vi "ArrangeFrontPanel.vi"(8 "error in (no error)":errorcluster, 10 "This VI":refnum<vi>, 11 "MAUI in":refnum<class "MAUI.lvclass">) -> (0 "error out":errorcluster, 3 "MAUI out":refnum<class "MAUI.lvclass">)   [LabVIEW 2019, in "MAUI.lvclass"]
doc: "This VI is mainly used for the MAUI Template. It will be removed from the library soon."
uses:
  MAUI.lvclass
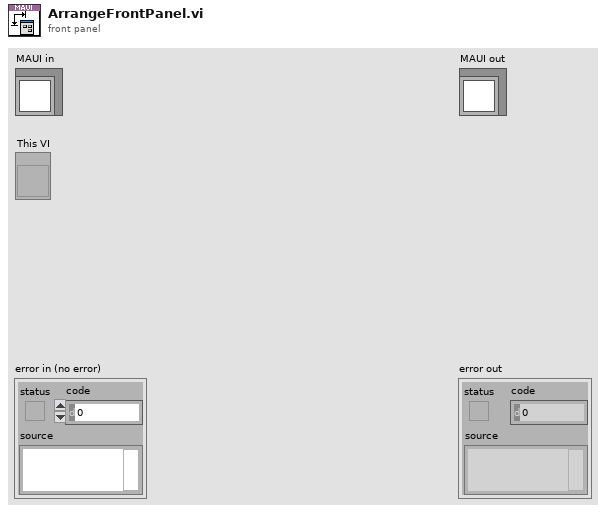
[diagram p1: front panel]
types:
  T1 = typedef "LVRectTypeDef.ctl" = cluster{"Left":i16, "Top":i16, "Right":i16, "Bottom":i16}
  T2 = typedef "LVBoundsTypeDef.ctl" = cluster{"Width":u32, "Height":u32}
  T3 = enum16{"Always On", "Always Off", "Off While Running"}
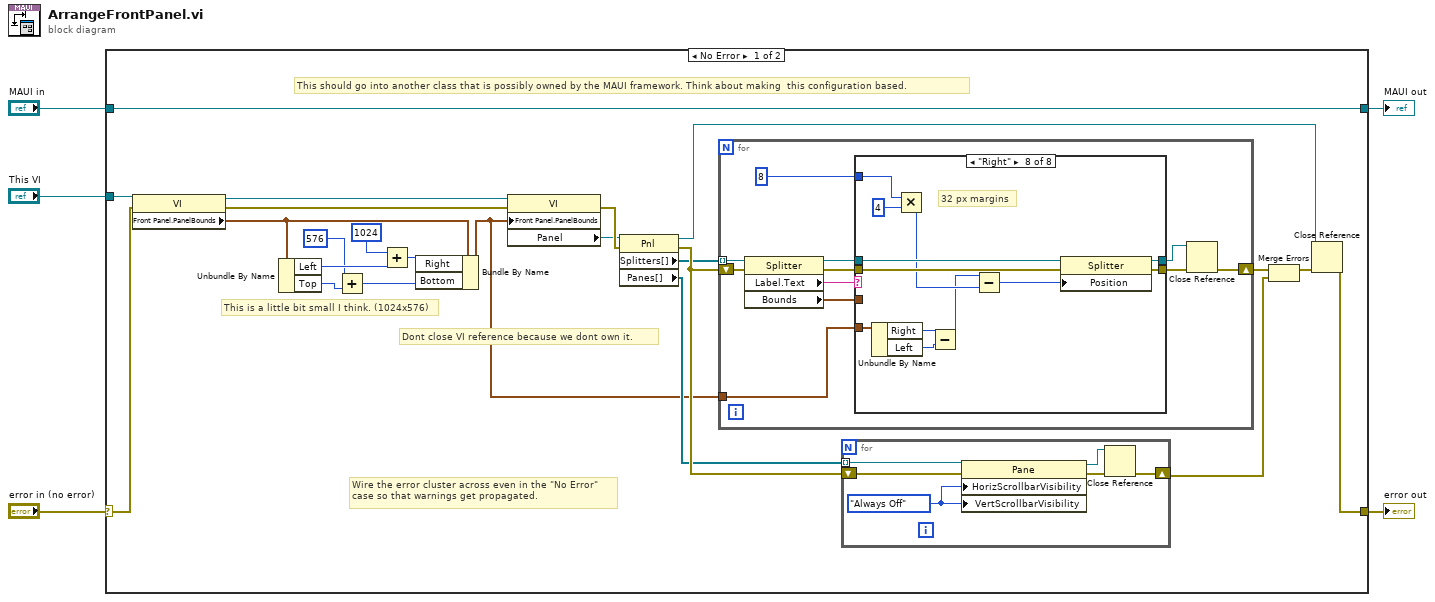
[diagram p0: block diagram]
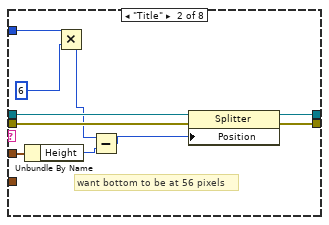
[diagram p3: hidden frame]
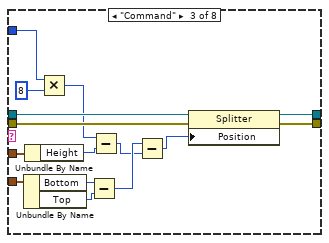
[diagram p4: hidden frame]
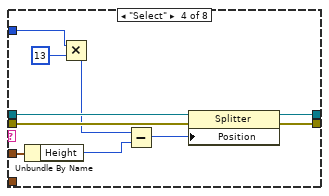
[diagram p5: hidden frame]
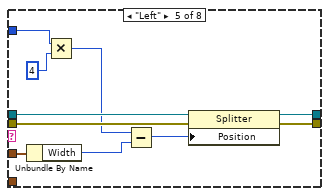
[diagram p6: hidden frame]
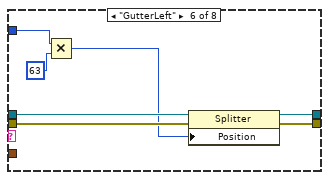
[diagram p7: hidden frame]
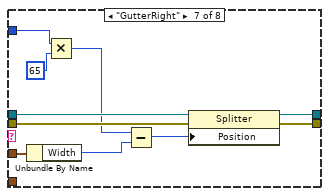
[diagram p8: hidden frame]
diagram:
  n1 = case shown="No Error" "error in (no error)" {
    selector: "error in (no error)" -> [w26 w123]
    tunnel: [w25 w123] -> w4
    tunnel: [w20 w122] -> w2
    tunnel: "MAUI in" -> [w20 w122]
    tunnel: "This VI" -> [w19 _]
    frame No Error {
      # "This should go into another class that is possibly owned by the MAUI framework. Think about making  this configuration based."
      # "This is a little bit small I think. (1024x576)"
      # "Dont close VI reference because we dont own it."
      # "Wire the error cluster across even in the \"No Error\"\ncase so that warnings get propagated."
      n2 = property on="Property Node" class="VI"(reference=w19, error in=w26) -> (reference out=w14:refnum<vi>, error out=w28:errorcluster, "Front Panel.PanelBounds"=w18:T1)
      n3 = Unbundle By Name(w18) -> ("Left"=w16:i16, "Top"=w7:i16)
      n4 = Add(x=i16 576, y=w7) -> (x+y=w17:i16)
      n5 = Add(x=i16 1024, y=w16) -> (x+y=w15:i16)
      n6 = Bundle By Name(cluster=w18, "Right"=w15, "Bottom"=w17) -> (w8:T1)
      n7 = property on="Property Node" class="VI"(reference=w14, error in=w28, "Front Panel.PanelBounds"=w8) -> (error out=w27:errorcluster, "Panel"=w13:refnum<vi>)  [unwired: 1 out]
      n8 = property on="Property Node" class="Pnl"(reference=w13, error in=w27) -> (reference out=w11:refnum<vi>, error out=w24:errorcluster, "Splitters[]"=w12:refnum<vi>[], "Panes[]"=w10:refnum<vi>[])
      n9 = for {
        tunnel: w12 -> [w41] mode=indexing
        shift-right: [w43] -> w23
        shift-left: w24 -> [w45]
        tunnel: w8 -> [w35]
        n10 = property on="Property Node" class="Splitter"(reference=w41, error in=w45) -> (reference out=w38:refnum<vi>, error out=w44:errorcluster, "Label.Text"=w40:string, "Bounds"=w39:T2)
        n11 = case shown="\"Right\"" w40 {
          tunnel: w44 -> [w47 w57 w72 w82 w92 w99 w109 w120]
          tunnel: w39 -> [_ w54 w69 w79 w89 _ w106 _]
          tunnel: [w47 w56 w71 w81 w91 w98 w108 w121] -> w42
          tunnel: w38 -> [w46 w55 w70 w80 w90 w97 w107 w118]
          tunnel: [w46 w51 w66 w77 w87 w96 w104 w119] -> w37
          tunnel: 8 -> [_ w50 w65 w75 w85 w95 w102 w117]
          tunnel: w35 -> [_ _ w63 _ _ _ _ w115]
          frame Default {
          }
          frame "Title" {
            # "want bottom to be at 56 pixels"
            n12 = Unbundle By Name(w54) -> ("Height"=w53:u32)
            n13 = Multiply(x=w50, y=6) -> (x*y=w48:i32)
            n14 = Subtract(x=w48, y=w53) -> (x-y=w52:u32)
            n15 = property on="Property Node" class="Splitter"(reference=w55, error in=w57, "Position"=w52) -> (reference out=w51:refnum<vi>, error out=w56:errorcluster)
          }
          frame "Command" {
            n16 = Unbundle By Name(w63) -> ("Bottom"=w62:i16, "Top"=w61:i16)
            n17 = Unbundle By Name(w69) -> ("Height"=w68:u32)
            n18 = Multiply(x=w65, y=8) -> (x*y=w67:i32)
            n19 = Subtract(x=w62, y=w61) -> (x-y=w59:i16)
            n20 = Subtract(x=w67, y=w68) -> (x-y=w58:u32)
            n21 = Subtract(x=w59, y=w58) -> (x-y=w60:u32)
            n22 = property on="Property Node" class="Splitter"(reference=w70, error in=w72, "Position"=w60) -> (reference out=w66:refnum<vi>, error out=w71:errorcluster)
          }
          frame "Select" {
            n23 = Unbundle By Name(w79) -> ("Height"=w76:u32)
            n24 = Multiply(x=w75, y=13) -> (x*y=w73:i32)
            n25 = Subtract(x=w73, y=w76) -> (x-y=w78:u32)
            n26 = property on="Property Node" class="Splitter"(reference=w80, error in=w82, "Position"=w78) -> (reference out=w77:refnum<vi>, error out=w81:errorcluster)
          }
          frame "Left" {
            n27 = Unbundle By Name(w89) -> ("Width"=w86:u32)
            n28 = Multiply(x=w85, y=4) -> (x*y=w83:i32)
            n29 = Subtract(x=w83, y=w86) -> (x-y=w88:u32)
            n30 = property on="Property Node" class="Splitter"(reference=w90, error in=w92, "Position"=w88) -> (reference out=w87:refnum<vi>, error out=w91:errorcluster)
          }
          frame "GutterLeft" {
            n31 = Multiply(x=w95, y=63) -> (x*y=w93:i32)
            n32 = property on="Property Node" class="Splitter"(reference=w97, error in=w99, "Position"=w93) -> (reference out=w96:refnum<vi>, error out=w98:errorcluster)
          }
          frame "GutterRight" {
            n33 = Unbundle By Name(w106) -> ("Width"=w103:u32)
            n34 = Multiply(x=w102, y=65) -> (x*y=w100:i32)
            n35 = Subtract(x=w100, y=w103) -> (x-y=w105:u32)
            n36 = property on="Property Node" class="Splitter"(reference=w107, error in=w109, "Position"=w105) -> (reference out=w104:refnum<vi>, error out=w108:errorcluster)
          }
          frame "Right" {
            # "32 px margins"
            n37 = Unbundle By Name(w115) -> ("Right"=w114:i16, "Left"=w113:i16)
            n38 = Multiply(x=w117, y=4) -> (x*y=w112:i32)
            n39 = Subtract(x=w114, y=w113) -> (x-y=w111:i16)
            n40 = Subtract(x=w111, y=w112) -> (x-y=w110:i32)
            n41 = property on="Property Node" class="Splitter"(reference=w118, error in=w120, "Position"=w110) -> (reference out=w119:refnum<vi>, error out=w121:errorcluster)
          }
        }
        n42 = Close Reference(reference=w37, error in (no error)=w42) -> (error out=w43:errorcluster)
      }
      n43 = for {
        tunnel: w10 -> [w31] mode=indexing
        shift-right: [w33] -> w21
        shift-left: w24 -> [w34]
        w29 = T3."Always Off" ("Horizontal Scrollbar Visibility")
        n44 = property on="Property Node" class="Pane"(reference=w31, error in=w34, "HorizScrollbarVisibility"=w29, "VertScrollbarVisibility"=w29) -> (reference out=w30:refnum<vi>, error out=w32:errorcluster)
        n45 = Close Reference(reference=w30, error in (no error)=w32) -> (error out=w33:errorcluster)
      }
      n46 = Merge Errors(w23, w21) -> (w22:errorcluster)
      n47 = Close Reference(reference=w11, error in (no error)=w22) -> (error out=w25:errorcluster)
    }
    frame Error {
    }
  }
  "error out" <- w4
  "MAUI out" <- w2
